vi "RichToFlatnixnet_grpc_TimeLocalNetwork.vi"(5 "OutputClusterType":T1, 11 "InputCluster":T2) -> (3 "OutputCluster":T1)   [LabVIEW 2025, in "xnet-grpc_client.lvlib"]
uses:
  nixnet_grpc_TimeLocalNetwork.ctl
  nixnet_grpc_TimeLocalNetwork_Flat.ctl
  xnet-grpc_client.lvlib
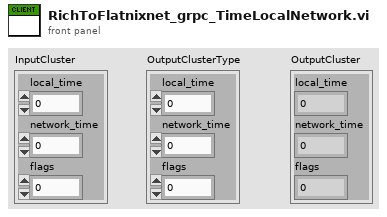
[diagram p1: front panel]
types:
  T1 = typedef "xnet-grpc_client.lvlib/nixnet_grpc_TimeLocalNetwork_Flat.ctl" = cluster{"local_time":u64, "network_time":u64, "flags":u32}
  T2 = typedef "xnet-grpc_client.lvlib/nixnet_grpc_TimeLocalNetwork.ctl" = cluster{"local_time":u64, "network_time":u64, "flags":u32}
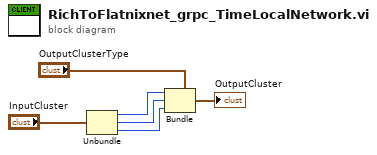
[diagram p0: block diagram]
diagram:
  n1 = Unbundle "Unbundle"("InputCluster") -> ("local_time"=w3:u64, "network_time"=w2:u64, "flags"=w1:u32)
  n2 = Bundle "Bundle"(cluster="OutputClusterType", "local_time"=w3, "network_time"=w2, "flags"=w1) -> (→"OutputCluster":T1)
